vi "数据索引起始时间填补空白.vi"(8 "error in (no error)":errorcluster caption="错误输入（无错误）") -> (0 "error out":errorcluster caption="错误输出")   [LabVIEW 2016, in "数据传输系统-02.lvlib"]
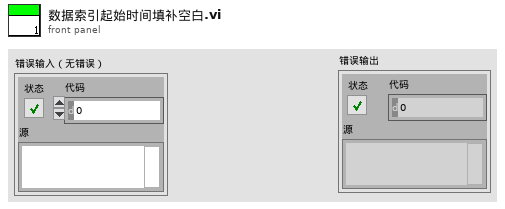
[diagram p1: front panel]
types:
  T1 = typedef "LVDateTimeRec.ctl" = cluster{"秒数的小数部分":dbl, "秒":i32, "分":i32, "时":i32, "日":i32, "月":i32, "年":i32, "天数（周）":i32, "天数（年）":i32, "DST":i32}
  T2 = cluster{"氨氮仪器参数索引起始时间":string, "总磷仪器参数索引起始时间":string, "总氮仪器参数索引起始时间":string, "CODMn仪器参数索引起始时间":string, "CODCr仪器参数索引起始时间":string, "DO仪器参数索引起始时间":string, "PH仪器参数索引起始时间":string, "比电导率仪器参数索引起始时间":string, "水温仪器参数索引起始时间":string, "浊度仪器参数索引起始时间":string, "叶绿素a仪器参数索引起始时间":string, "藻密度仪器参数索引起始时间":string, "ORP仪器参数索引起始时间":string, "氟化物仪器参数索引起始时间":string}
  T3 = cluster{"氨氮加标回收索引起始时间":string, "总磷加标回收索引起始时间":string, "总氮加标回收索引起始时间":string, "CODMn加标回收索引起始时间":string, "CODCr加标回收索引起始时间":string, "氟化物加标回收索引起始时间":string}
  T4 = cluster{"氨氮跨度核查索引起始时间":string, "总磷跨度核查索引起始时间":string, "总氮跨度核查索引起始时间":string, "CODMn跨度核查索引起始时间":string, "CODCr跨度核查索引起始时间":string, "亚硝酸盐跨度核查索引起始时间":string, "硫化物跨度核查索引起始时间":string, "ORP跨度核查索引起始时间":string, "氟化物跨度核查索引起始时间":string}
  T5 = cluster{"氨氮零点核查索引起始时间":string, "总磷零点核查索引起始时间":string, "总氮零点核查索引起始时间":string, "CODMn零点核查索引起始时间":string, "CODCr零点核查索引起始时间":string, "亚硝酸盐零点核查索引起始时间":string, "硫化物零点核查索引起始时间":string, "ORP零点核查索引起始时间":string, "氟化物零点核查索引起始时间":string}
  T6 = cluster{"氨氮报警信息索引起始时间":string, "总磷报警信息索引起始时间":string, "总氮报警信息索引起始时间":string, "CODMn报警信息索引起始时间":string, "CODCr报警信息索引起始时间":string, "DO报警信息索引起始时间":string, "PH报警信息索引起始时间":string, "比电导率报警信息索引起始时间":string, "水温报警信息索引起始时间":string, "浊度报警信息索引起始时间":string, "叶绿素报警信息索引起始时间":string, "系统报警信息索引起始时间":string, "氟化物报警信息索引起始时间":string}
  T7 = cluster{"氨氮标样核查索引起始时间":string, "总磷标样核查索引起始时间":string, "总氮标样核查索引起始时间":string, "CODMn标样核查索引起始时间":string, "CODCr标样核查索引起始时间":string, "DO标样核查索引起始时间":string, "PH标样核查索引起始时间":string, "比电导率标样核查索引起始时间":string, "水温标样核查索引起始时间":string, "浊度标样核查索引起始时间":string, "叶绿素a标样核查索引起始时间":string, "藻密度标样核查索引起始时间":string, "亚硝酸盐标样核查索引起始时间":string, "硫化物标样核查索引起始时间":string, "ORP标样核查索引起始时间":string, "氟化物标样核查索引起始时间":string}
  T8 = cluster{"氨氮集成干预索引起始时间":string, "总磷集成干预索引起始时间":string, "总氮集成干预索引起始时间":string, "CODMn集成干预索引起始时间":string, "CODCr集成干预索引起始时间":string, "DO集成干预索引起始时间":string, "PH集成干预索引起始时间":string, "比电导率集成干预索引起始时间":string, "水温集成干预索引起始时间":string, "浊度集成干预索引起始时间":string, "叶绿素a集成干预索引起始时间":string, "藻密度集成干预索引起始时间":string, "亚硝酸盐集成干预索引起始时间":string, "硫化物集成干预索引起始时间":string, "ORP集成干预索引起始时间":string, "氟化物集成干预索引起始时间":string}
  T9 = cluster{"氨氮仪器日志索引起始时间":string, "总磷仪器日志索引起始时间":string, "总氮仪器日志索引起始时间":string, "CODMn仪器日志索引起始时间":string, "CODCr仪器日志索引起始时间":string, "系统仪器日志索引起始时间":string, "氟化物仪器日志索引起始时间":string}
  T10 = cluster{"氨氮平行样索引起始时间":string, "总磷平行样索引起始时间":string, "总氮平行样索引起始时间":string, "CODMn平行样索引起始时间":string, "CODCr平行样索引起始时间":string, "氟化物平行样索引起始时间":string}
  T11 = cluster{"[0]":string, "[1]":string, "[2]":string, "[3]":string, "[4]":string, "[5]":string}
  T12 = cluster{"[0]":string, "[1]":string, "[2]":string, "[3]":string, "[4]":string, "[5]":string, "[6]":string, "[7]":string, "[8]":string}
  T13 = cluster{"[0]":string, "[1]":string, "[2]":string, "[3]":string, "[4]":string, "[5]":string, "[6]":string, "[7]":string, "[8]":string, "[9]":string, "[10]":string, "[11]":string, "[12]":string}
  T14 = cluster{"[0]":string, "[1]":string, "[2]":string, "[3]":string, "[4]":string, "[5]":string, "[6]":string, "[7]":string, "[8]":string, "[9]":string, "[10]":string, "[11]":string, "[12]":string, "[13]":string, "[14]":string, "[15]":string}
  T15 = cluster{"[0]":string, "[1]":string, "[2]":string, "[3]":string, "[4]":string, "[5]":string, "[6]":string, "[7]":string, "[8]":string, "[9]":string, "[10]":string, "[11]":string, "[12]":string, "[13]":string}
  T16 = cluster{"[0]":string, "[1]":string, "[2]":string, "[3]":string, "[4]":string, "[5]":string, "[6]":string}
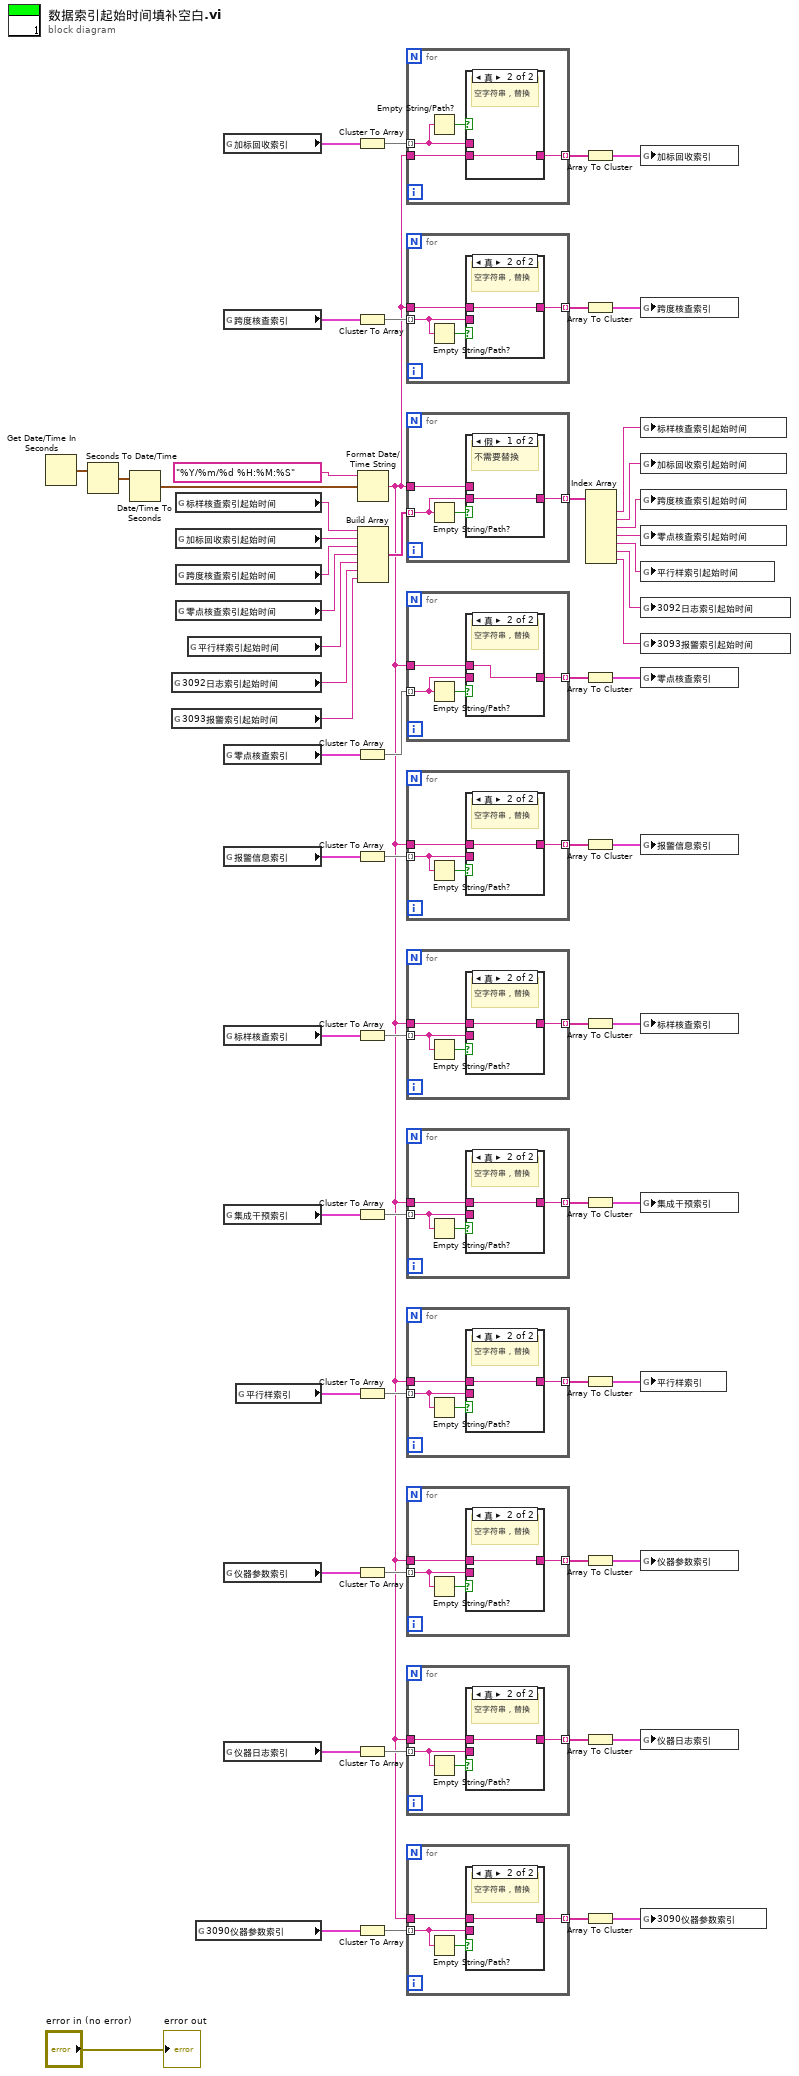
[diagram p0: block diagram]
diagram:
  n1 = Get Date/Time In Seconds() -> (seconds since 1Jan1904=w62:timestamp)
  n2 = Seconds To Date/Time(time stamp (now)=w62) -> (date time rec=w60:T1)  [unwired: 1 in]
  n3 = Date/Time To Seconds(2:w60) -> (0:w59:timestamp)  [unwired: 1 in]
  n4 = global read "全局 时间2.vi" "3092日志索引起始时间"() -> (w4:string)
  n5 = global read "全局 时间2.vi" "3093报警索引起始时间"() -> (w2:string)
  n6 = global read "全局 时间2.vi" "标样核查索引起始时间"() -> (w25:string)
  n7 = global read "全局 时间2.vi" "加标回收索引起始时间"() -> (w24:string)
  n8 = global read "全局 时间2.vi" "跨度核查索引起始时间"() -> (w23:string)
  n9 = global read "全局 时间2.vi" "零点核查索引起始时间"() -> (w21:string)
  n10 = global read "全局 时间2.vi" "平行样索引起始时间"() -> (w22:string)
  n11 = global read "全局 时间2.vi" "3090仪器参数索引"() -> (w13:T2)
  n12 = global read "全局 时间2.vi" "加标回收索引"() -> (w9:T3)
  n13 = global read "全局 时间2.vi" "跨度核查索引"() -> (w39:T4)
  n14 = global read "全局 时间2.vi" "零点核查索引"() -> (w58:T5)
  n15 = global read "全局 时间2.vi" "报警信息索引"() -> (w51:T6)
  n16 = global read "全局 时间2.vi" "标样核查索引"() -> (w50:T7)
  n17 = global read "全局 时间2.vi" "集成干预索引"() -> (w43:T8)
  n18 = global read "全局 时间2.vi" "仪器参数索引"() -> (w31:T2)
  n19 = global read "全局 时间2.vi" "仪器日志索引"() -> (w30:T9)
  n20 = global read "全局 时间2.vi" "平行样索引"() -> (w38:T10)
  n21 = Cluster To Array(cluster=w9) -> (array=w8:string[])
  n22 = Cluster To Array(cluster=w39) -> (array=w40:string[])
  n23 = Cluster To Array(cluster=w58) -> (array=w57:string[])
  n24 = Cluster To Array(cluster=w51) -> (array=w52:string[])
  n25 = Cluster To Array(cluster=w50) -> (array=w49:string[])
  n26 = Cluster To Array(cluster=w43) -> (array=w44:string[])
  n27 = Cluster To Array(cluster=w38) -> (array=w37:string[])
  n28 = Cluster To Array(cluster=w31) -> (array=w32:string[])
  n29 = Cluster To Array(cluster=w30) -> (array=w29:string[])
  n30 = Cluster To Array(cluster=w13) -> (array=w12:string[])
  n31 = Format Date/Time String(time format string (%c)="%Y/%m/%d %H:%M:%S" ("时间格式字符串(%c)"), seconds (now)=w59) -> (date/time string=w5:string)  [unwired: 1 in]
  n32 = Build Array(w25, w24, w23, w21, w22, w4, w2) -> (w20:string[])
  n33 = for {
    tunnel: w8 -> [w63] mode=indexing
    tunnel: w5 -> [w65]
    tunnel: [w64] -> w7 mode=indexing
    n34 = Empty String/Path?(string/path=w63) -> (empty?=w66:bool)
    n35 = case shown="真" w66 {
      tunnel: w65 -> [_ w68]
      tunnel: [w67 w68] -> w64
      tunnel: w63 -> [w67 _]
      frame False {
        # "不需要替换"
      }
      frame True {
        # "空字符串，替换"
      }
    }
  }
  n36 = for {
    tunnel: w40 -> [w69] mode=indexing
    tunnel: w5 -> [w71]
    tunnel: [w70] -> w41 mode=indexing
    n37 = Empty String/Path?(string/path=w69) -> (empty?=w72:bool)
    n38 = case shown="真" w72 {
      tunnel: w71 -> [_ w74]
      tunnel: [w73 w74] -> w70
      tunnel: w69 -> [w73 _]
      frame False {
        # "不需要替换"
      }
      frame True {
        # "空字符串，替换"
      }
    }
  }
  n39 = for {
    tunnel: w20 -> [w76] mode=indexing
    tunnel: w5 -> [w77]
    tunnel: [w75] -> w19 mode=indexing
    n40 = Empty String/Path?(string/path=w76) -> (empty?=w78:bool)
    n41 = case shown="假" w78 {
      tunnel: w77 -> [_ w80]
      tunnel: [w79 w80] -> w75
      tunnel: w76 -> [w79 _]
      frame False {
        # "不需要替换"
      }
      frame True {
        # "空字符串，替换"
      }
    }
  }
  n42 = for {
    tunnel: w57 -> [w81] mode=indexing
    tunnel: w5 -> [w83]
    tunnel: [w82] -> w56 mode=indexing
    n43 = Empty String/Path?(string/path=w81) -> (empty?=w84:bool)
    n44 = case shown="真" w84 {
      tunnel: w83 -> [_ w86]
      tunnel: [w85 w86] -> w82
      tunnel: w81 -> [w85 _]
      frame False {
        # "不需要替换"
      }
      frame True {
        # "空字符串，替换"
      }
    }
  }
  n45 = for {
    tunnel: w52 -> [w87] mode=indexing
    tunnel: w5 -> [w89]
    tunnel: [w88] -> w53 mode=indexing
    n46 = Empty String/Path?(string/path=w87) -> (empty?=w90:bool)
    n47 = case shown="真" w90 {
      tunnel: w89 -> [_ w92]
      tunnel: [w91 w92] -> w88
      tunnel: w87 -> [w91 _]
      frame False {
        # "不需要替换"
      }
      frame True {
        # "空字符串，替换"
      }
    }
  }
  n48 = for {
    tunnel: w49 -> [w93] mode=indexing
    tunnel: w5 -> [w95]
    tunnel: [w94] -> w48 mode=indexing
    n49 = Empty String/Path?(string/path=w93) -> (empty?=w96:bool)
    n50 = case shown="真" w96 {
      tunnel: w95 -> [_ w98]
      tunnel: [w97 w98] -> w94
      tunnel: w93 -> [w97 _]
      frame False {
        # "不需要替换"
      }
      frame True {
        # "空字符串，替换"
      }
    }
  }
  n51 = for {
    tunnel: w44 -> [w99] mode=indexing
    tunnel: w5 -> [w101]
    tunnel: [w100] -> w45 mode=indexing
    n52 = Empty String/Path?(string/path=w99) -> (empty?=w102:bool)
    n53 = case shown="真" w102 {
      tunnel: w101 -> [_ w104]
      tunnel: [w103 w104] -> w100
      tunnel: w99 -> [w103 _]
      frame False {
        # "不需要替换"
      }
      frame True {
        # "空字符串，替换"
      }
    }
  }
  n54 = for {
    tunnel: w37 -> [w105] mode=indexing
    tunnel: w5 -> [w107]
    tunnel: [w106] -> w36 mode=indexing
    n55 = Empty String/Path?(string/path=w105) -> (empty?=w108:bool)
    n56 = case shown="真" w108 {
      tunnel: w107 -> [_ w110]
      tunnel: [w109 w110] -> w106
      tunnel: w105 -> [w109 _]
      frame False {
        # "不需要替换"
      }
      frame True {
        # "空字符串，替换"
      }
    }
  }
  n57 = for {
    tunnel: w32 -> [w111] mode=indexing
    tunnel: w5 -> [w113]
    tunnel: [w112] -> w33 mode=indexing
    n58 = Empty String/Path?(string/path=w111) -> (empty?=w114:bool)
    n59 = case shown="真" w114 {
      tunnel: w113 -> [_ w116]
      tunnel: [w115 w116] -> w112
      tunnel: w111 -> [w115 _]
      frame False {
        # "不需要替换"
      }
      frame True {
        # "空字符串，替换"
      }
    }
  }
  n60 = for {
    tunnel: w29 -> [w117] mode=indexing
    tunnel: w5 -> [w119]
    tunnel: [w118] -> w28 mode=indexing
    n61 = Empty String/Path?(string/path=w117) -> (empty?=w120:bool)
    n62 = case shown="真" w120 {
      tunnel: w119 -> [_ w122]
      tunnel: [w121 w122] -> w118
      tunnel: w117 -> [w121 _]
      frame False {
        # "不需要替换"
      }
      frame True {
        # "空字符串，替换"
      }
    }
  }
  n63 = for {
    tunnel: w12 -> [w123] mode=indexing
    tunnel: w5 -> [w125]
    tunnel: [w124] -> w11 mode=indexing
    n64 = Empty String/Path?(string/path=w123) -> (empty?=w126:bool)
    n65 = case shown="真" w126 {
      tunnel: w125 -> [_ w128]
      tunnel: [w127 w128] -> w124
      tunnel: w123 -> [w127 _]
      frame False {
        # "不需要替换"
      }
      frame True {
        # "空字符串，替换"
      }
    }
  }
  n66 = Array To Cluster(array=w7) -> (cluster=w6:T11)
  n67 = Array To Cluster(array=w41) -> (cluster=w42:T12)
  n68 = Array To Cluster(array=w56) -> (cluster=w55:T12)
  n69 = Array To Cluster(array=w53) -> (cluster=w54:T13)
  n70 = Array To Cluster(array=w48) -> (cluster=w47:T14)
  n71 = Array To Cluster(array=w45) -> (cluster=w46:T14)
  n72 = Array To Cluster(array=w36) -> (cluster=w35:T11)
  n73 = Array To Cluster(array=w33) -> (cluster=w34:T15)
  n74 = Array To Cluster(array=w28) -> (cluster=w27:T16)
  n75 = Array To Cluster(array=w11) -> (cluster=w10:T15)
  n76 = Index Array(array=w19) -> (element #1=w18:string, element #2=w17:string, element #3=w16:string, element #4=w14:string, element #5=w15:string, element #6=w3:string, element #7=w1:string)  [unwired: 7 in]
  n77 = global write "全局 时间2.vi" "加标回收索引"(w6) -> ()
  n78 = global write "全局 时间2.vi" "跨度核查索引"(w42) -> ()
  n79 = global write "全局 时间2.vi" "标样核查索引起始时间"(w18) -> ()
  n80 = global write "全局 时间2.vi" "加标回收索引起始时间"(w17) -> ()
  n81 = global write "全局 时间2.vi" "跨度核查索引起始时间"(w16) -> ()
  n82 = global write "全局 时间2.vi" "零点核查索引起始时间"(w14) -> ()
  n83 = global write "全局 时间2.vi" "平行样索引起始时间"(w15) -> ()
  n84 = global write "全局 时间2.vi" "3092日志索引起始时间"(w3) -> ()
  n85 = global write "全局 时间2.vi" "3093报警索引起始时间"(w1) -> ()
  n86 = global write "全局 时间2.vi" "零点核查索引"(w55) -> ()
  n87 = global write "全局 时间2.vi" "报警信息索引"(w54) -> ()
  n88 = global write "全局 时间2.vi" "标样核查索引"(w47) -> ()
  n89 = global write "全局 时间2.vi" "集成干预索引"(w46) -> ()
  n90 = global write "全局 时间2.vi" "平行样索引"(w35) -> ()
  n91 = global write "全局 时间2.vi" "仪器参数索引"(w34) -> ()
  n92 = global write "全局 时间2.vi" "仪器日志索引"(w27) -> ()
  n93 = global write "全局 时间2.vi" "3090仪器参数索引"(w10) -> ()
  "error out" <- "error in (no error)"
